vi "Write Database.vi"(8 "error in (no error)":errorcluster, 10 "Database":refnum<class "Database Adv Schema.lvclass">, 11 "Table Configuration Adv Schema DB in":refnum<class "Table Configuration Adv Schema DB.lvclass">) -> (0 "error out":errorcluster, 3 "Table Configuration Adv Schema DB out":refnum<class "Table Configuration Adv Schema DB.lvclass">)   [LabVIEW 2020, in "Table.lvlib" / "Table Configuration Adv Schema DB.lvclass"]
uses:
  Table Configuration Adv Schema DB.lvclass
  Database Libraries/Database Interfaces/Database Advanced Schema Class/Database Adv Schema.lvclass
  Table Configuration Adv Schema DB.lvclass/Table Configuration Adv Schema DB.ctl
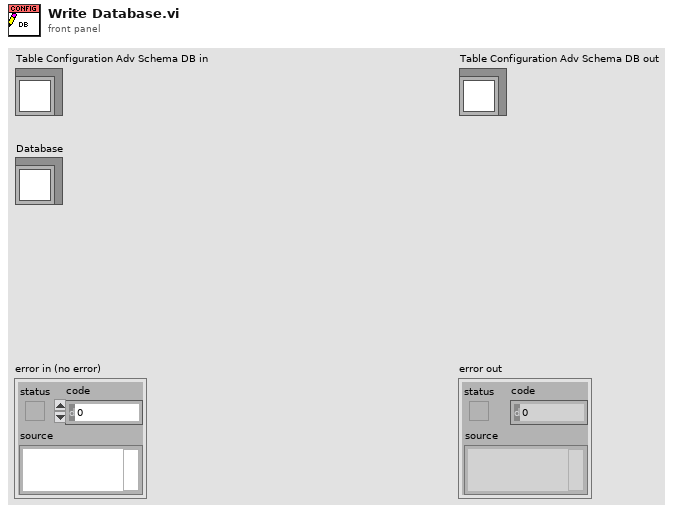
[diagram p1: front panel]
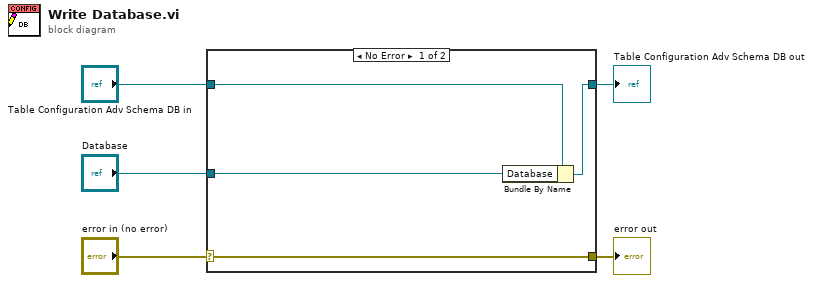
[diagram p0: block diagram]
diagram:
  n1 = case shown="No Error" "error in (no error)" {
    selector: "error in (no error)" -> [w9 w10]
    tunnel: [w9 w10] -> w4
    tunnel: [w7 w11] -> w2
    tunnel: "Table Configuration Adv Schema DB in" -> [w8 w11]
    tunnel: "Database" -> [w6 _]
    frame No Error {
      n2 = Bundle By Name(cluster=w8, "Database"=w6) -> (w7:refnum<class "Table Configuration Adv Schema DB.lvclass">)
    }
    frame Error {
    }
  }
  "error out" <- w4
  "Table Configuration Adv Schema DB out" <- w2
